vi "Write Plot Info.vi"(5 "Plot Info":T1, 9 "Plot in":refnum<class "Plot.lvclass">) -> (3 "Plot out":refnum<class "Plot.lvclass">)   [LabVIEW 2014, in "Plot.lvclass"]
uses:
  Plot.lvclass
  Plot.lvclass/Plot.ctl
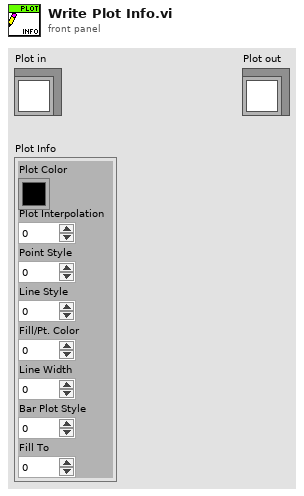
[diagram p1: front panel]
types:
  T1 = cluster{"Plot Color":u32, "Plot Interpolation":u8, "Point Style":u8, "Line Style":u8, "Fill/Pt. Color":u32, "Line Width":u8, "Bar Plot Style":u8, "Fill To":i16}
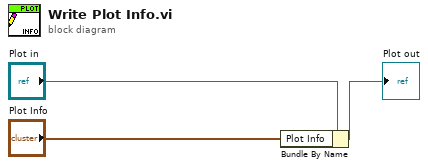
[diagram p0: block diagram]
diagram:
  n1 = Bundle By Name(cluster="Plot in", "Plot Info"="Plot Info") -> (→"Plot out":refnum<class "Plot.lvclass">)
